vi "Configure Output Amplifier.vi"(8 "error in (no error)":errorcluster, 9 "Amplifier Type (0: Maximum Amplitude)":i32(ring) items=["Maximum Amplitude", "Maximum Bandwidth"], 10 "Channel (1: Channel1)":u16(ring) items=["Channel1", "Channel2"], 11 "VISA resource name":refnum<visa-resource-name>) -> (0 "error out":errorcluster, 3 "VISA resource name out":refnum<visa-resource-name>)   [LabVIEW 2009, in "Agilent 81150.lvlib"]
doc: "Configures the amplifier type."
uses:
  Agilent 81150.lvlib
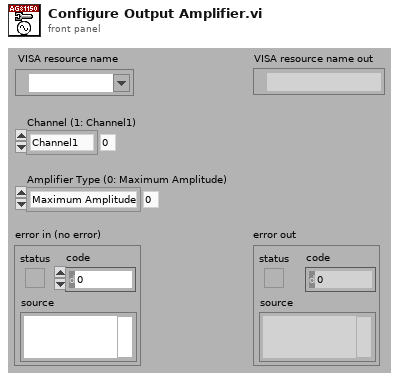
[diagram p1: front panel]
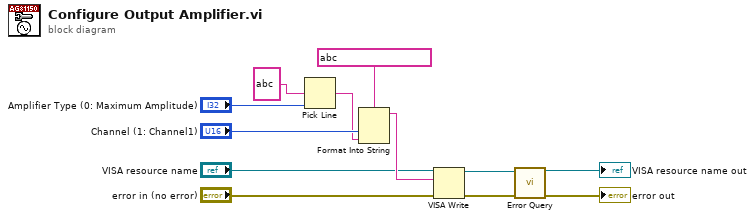
[diagram p0: block diagram]
diagram:
  n1 = Pick Line(multi-line string=string ?, line index="Amplifier Type (0: Maximum Amplitude)") -> (output string=w8:string)  [unwired: 1 out]
  n2 = Format Into String(format string=string ?, "Channel (1: Channel1)", w8) -> (resulting string=w7:string)  [unwired: 2 in, 1 out]
  n3 = VISA Write(VISA resource name="VISA resource name", write buffer=w7, error in (no error)="error in (no error)") -> (VISA resource name out=w4:refnum<visa-resource-name>, error out=w3:errorcluster)  [unwired: 1 out]
  n4 = call "Error Query.vi"("error in (no error)"=w3, "VISA resource name"=w4) -> ("error out"=→"error out":errorcluster, "VISA resource name out"=→"VISA resource name out":refnum<visa-resource-name>)  [unwired: 8 out]
